vi "Sync Ch TR Edge.vi"(7 "RxEdge":u8, 9 "TxEdge":u8, 10 "Channel":u8, 11 "devId":i32) -> (2 "devId out":i32, 3 "function return":i32)   [LabVIEW 2013, in "CHR34XXX.lvlib"]
doc: "DLL BOOL __stdcall CHR34XXX_Sync_Ch_LocalAddr(IN int devId,IN BYTE Channel,IN BYTE LocalAddr); DLL BOOL __stdcall CHR34XXX_Sync_Ch_SetCrc(IN int devId,IN BYTE Channel,IN BYTE CrcVal,IN BYTE CrcOrder); DLL BOOL __stdcall CHR34XXX_Sync_Ch_FrmId(IN int devId,IN BYTE Channel,IN WORD IdCnt,IN WORD IdPos,IN WORD IdOrder); DLL BOOL __stdcall CHR34XXX_Sync_Ch_MonitorEn(IN int devId,IN BYTE Channel,IN BOOL Enabled); DLL BOOL __stdcall CHR34XXX_Sync_Ch_TREdge(IN int devId,IN BYTE Channel,IN BYTE TxEdge,IN BYTE RxEdge);"
uses:
  CHR34XXX.lvlib
  CHR34XXX.dll
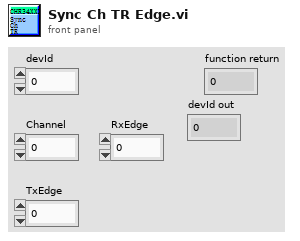
[diagram p1: front panel]
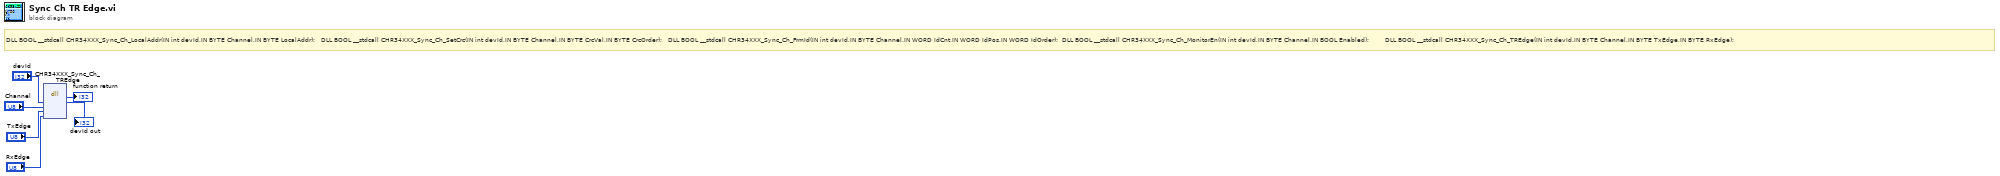
[diagram p0: block diagram]
diagram:
  # "DLL BOOL __stdcall CHR34XXX_Sync_Ch_LocalAddr(IN int devId,IN BYTE Channel,IN BYTE LocalAddr);   DLL BOOL __stdcall CHR34XXX_Sync_Ch_SetCrc(IN int devId,IN BYTE Channel,IN BYTE CrcVal,IN BYTE CrcOrder);   DLL BOOL __stdcall CHR34XXX_Sync_Ch_FrmId(IN int devId,IN BYTE Channel,IN WORD IdCnt,IN WORD IdPos,IN WORD IdOrder);  DLL BOOL __stdcall CHR34XXX_Sync_Ch_MonitorEn(IN int devId,IN BYTE Channel,IN BOOL Enabled);        DLL BOOL __stdcall CHR34XXX_Sync_Ch_TREdge(IN int devId,IN BYTE Channel,IN BYTE TxEdge,IN BYTE RxEdge);"
  n1 = dll-call lib="C:/Users/Administrator/Desktop/CHR34XXX_lv/lv_lib/CHR34XXX.*" fn="CHR34XXX_Sync_Ch_TREdge"("devId"="devId", "Channel"="Channel", "TxEdge"="TxEdge", "RxEdge"="RxEdge") -> (→"function return":i32, "devId"=→"devId out":i32)  [unwired: 6 in, 2 out]
